vi "GPIB_func.vi"(8 "error in (no error)":errorcluster, 9 "write buffer":string, 10 "Enum":T1(ring), 11 "VISA resource name":refnum<visa-resource-name>) -> (0 "error out":errorcluster, 3 "read buffer":string)   [LabVIEW 2015]
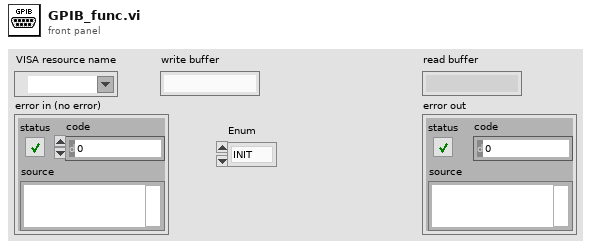
[diagram p1: front panel]
types:
  T1 = enum16{"INIT", "READ", "WRITE", "Query", "CLOSE"}
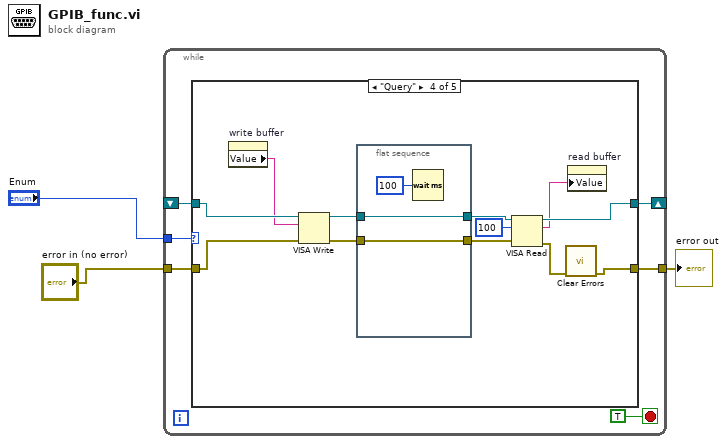
[diagram p0: block diagram]
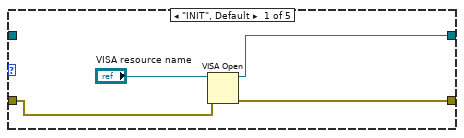
[diagram p2: hidden frame]
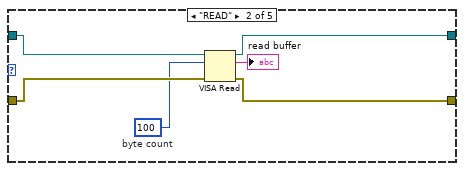
[diagram p3: hidden frame]
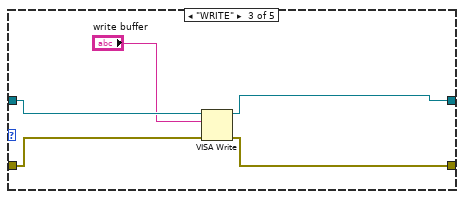
[diagram p4: hidden frame]
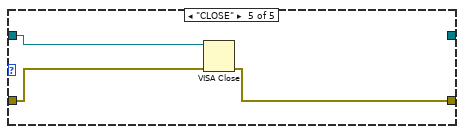
[diagram p5: hidden frame]
diagram:
  n1 = while {
    tunnel: "Enum" -> [w9]
    shift-right: [w7] -> _
    shift-left: _ -> [w6]
    tunnel: [w5] -> w1
    tunnel: "error in (no error)" -> [w4]
    stop <- TRUE stop-if-true
    n2 = case shown="\"Query\"" w9 {
      tunnel: [w12 w18 w23 w29 _] -> w7
      tunnel: w6 -> [_ w19 w24 w36 w40]
      tunnel: [w11 w16 w21 w26 w41] -> w5
      tunnel: w4 -> [w10 w17 w22 w35 w42]
      frame "INIT", Default {
        n3 = VISA Open(error in (no error)=w10, VISA resource name="VISA resource name") -> (VISA resource name=w12:refnum<visa-resource-name>, error out=w11:errorcluster)  [unwired: 3 in]
      }
      frame "READ" {
        w14 = u32 100  # byte count
        n4 = VISA Read(VISA resource name=w19, byte count=w14, error in (no error)=w17) -> (VISA resource name out=w18:refnum<visa-resource-name>, read buffer=→"read buffer":string, error out=w16:errorcluster)  [unwired: 1 out]
      }
      frame "WRITE" {
        n5 = VISA Write(VISA resource name=w24, write buffer="write buffer", error in (no error)=w22) -> (VISA resource name out=w23:refnum<visa-resource-name>, error out=w21:errorcluster)  [unwired: 1 out]
      }
      frame "Query" {
        n6 = property on="write buffer" class="Str"() -> ("Value"=w34:string)  [unwired: 2 in, 2 out]
        n7 = VISA Write(VISA resource name=w36, write buffer=w34, error in (no error)=w35) -> (VISA resource name out=w30:refnum<visa-resource-name>, error out=w33:errorcluster)  [unwired: 1 out]
        n8 = flat-sequence {
          tunnel: w33 -> [w39]
          tunnel: [w39] -> w32
          tunnel: [w38] -> w31
          tunnel: w30 -> [w38]
          frame #0 {
            n9 = Wait (ms)(milliseconds to wait=u32 100) -> ()  [unwired: 1 out]
          }
        }
        n10 = VISA Read(VISA resource name=w31, byte count=u32 100, error in (no error)=w32) -> (VISA resource name out=w29:refnum<visa-resource-name>, read buffer=w28:string, error out=w25:errorcluster)  [unwired: 1 out]
        n11 = call <vilib>:"Clear Errors.vi"("error in (no error)"=w25) -> ("error out"=w26:errorcluster)  [unwired: 5 in, 1 out]
        n12 = property on="read buffer" class="Str"("Value"=w28) -> ()  [unwired: 2 in, 2 out]
      }
      frame "CLOSE" {
        n13 = VISA Close(VISA resource name=w40, error in (no error)=w42) -> (error out=w41:errorcluster)
      }
    }
  }
  "error out" <- w1
